vi "configureConnectorPane.vi"(8 "error in (no error)":errorcluster, 11 "PolymorphicInstance in":refnum<class "PolymorphicInstance.lvclass">) -> (0 "error out":errorcluster, 3 "PolymorphicInstance out":refnum<class "PolymorphicInstance.lvclass">)   [LabVIEW 2012, in "PolymorphicInstance.lvclass"]
uses:
  PolymorphicInstance.lvclass
  PolymorphicInstance.lvclass/PolymorphicInstance.ctl
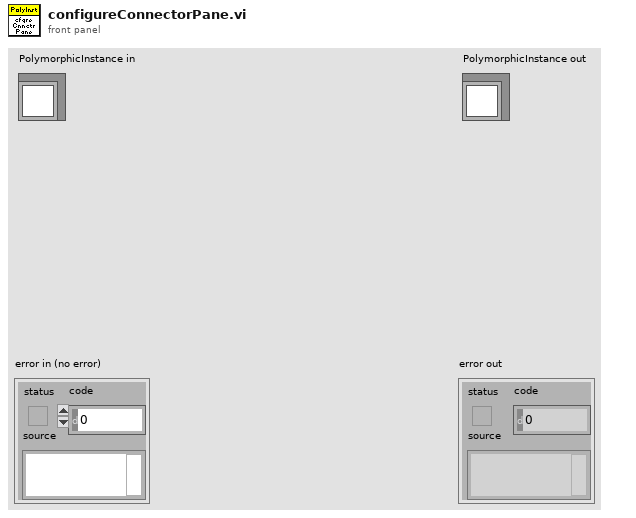
[diagram p1: front panel]
types:
  T1 = enum16{"Invalid Wire Rule", "Required", "Recommended", "Optional", "Dynamic Dispatch"}
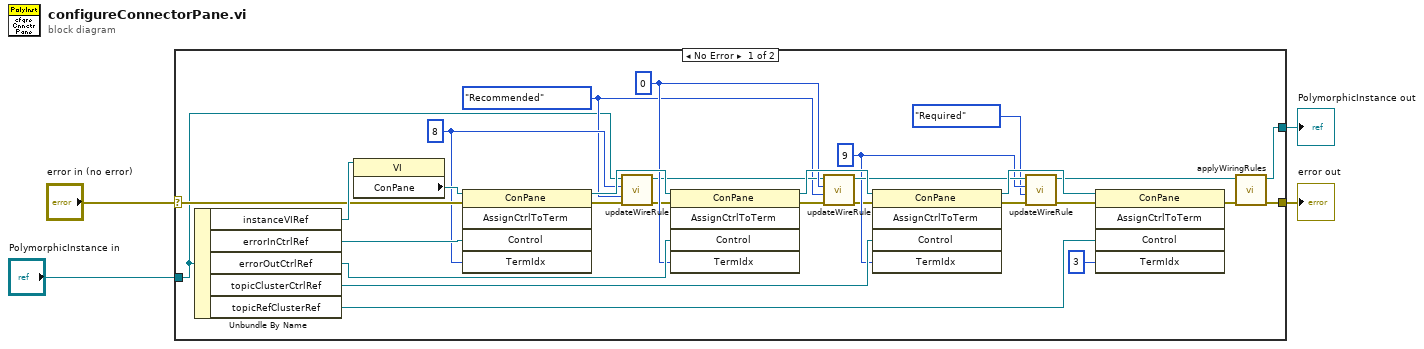
[diagram p0: block diagram]
diagram:
  n1 = case shown="No Error" "error in (no error)" {
    selector: "error in (no error)" -> [w30 w35]
    tunnel: [w14 w35] -> w3
    tunnel: [w12 w34] -> w1
    tunnel: "PolymorphicInstance in" -> [w15 w34]
    frame No Error {
      w19 = T1."Recommended" ("Wire Rule")
      w17 = u32 9 ("Terminal Index")
      w21 = u32 0 ("Terminal Index")
      w22 = u32 8 ("Terminal Index")
      n2 = Unbundle By Name(w15) -> ("instanceVIRef"=w33:refnum<vi>, "errorInCtrlRef"=w31:refnum<vi>, "errorOutCtrlRef"=w29:refnum<vi>, "topicClusterCtrlRef"=w24:refnum<vi>, "topicRefClusterRef"=w23:refnum<vi>)
      n3 = property class="VI"(reference=w33) -> ("ConPane"=w32:refnum<vi>)  [unwired: 1 in, 2 out]
      n4 = invoke class="ConPane" method="AssignCtrlToTerm"(reference=w32, error in=w30, "Control"=w31, "TermIdx"=w22) -> (reference out=w28:refnum<vi>, error out=w11:errorcluster)  [unwired: 1 in, 3 out]
      n5 = call "updateWireRule.vi"("error in (no error)"=w11, "Wire Rule"=w19, "terminalIndex"=w22, "PolymorphicInstance in"=w15) -> ("error out"=w10:errorcluster, "PolymorphicInstance out"=w20:refnum<class "PolymorphicInstance.lvclass">)  [unwired: 6 in]
      n6 = invoke class="ConPane" method="AssignCtrlToTerm"(reference=w28, error in=w10, "Control"=w29, "TermIdx"=w21) -> (reference out=w26:refnum<vi>, error out=w9:errorcluster)  [unwired: 1 in, 3 out]
      n7 = call "updateWireRule.vi"("error in (no error)"=w9, "Wire Rule"=w19, "terminalIndex"=w21, "PolymorphicInstance in"=w20) -> ("error out"=w8:errorcluster, "PolymorphicInstance out"=w18:refnum<class "PolymorphicInstance.lvclass">)  [unwired: 6 in]
      n8 = invoke class="ConPane" method="AssignCtrlToTerm"(reference=w26, error in=w8, "Control"=w24, "TermIdx"=w17) -> (reference out=w25:refnum<vi>, error out=w7:errorcluster)  [unwired: 1 in, 3 out]
      n9 = call "updateWireRule.vi"("error in (no error)"=w7, "Wire Rule"=T1."Required", "terminalIndex"=w17, "PolymorphicInstance in"=w18) -> ("error out"=w6:errorcluster, "PolymorphicInstance out"=w13:refnum<class "PolymorphicInstance.lvclass">)  [unwired: 6 in]
      n10 = invoke class="ConPane" method="AssignCtrlToTerm"(reference=w25, error in=w6, "Control"=w23, "TermIdx"=u32 3 ("Terminal Index")) -> (error out=w5:errorcluster)  [unwired: 1 in, 4 out]
      n11 = call "applyWiringRules.vi"("error in (no error)"=w5, "PolymorphicInstance in"=w13) -> ("error out"=w14:errorcluster, "PolymorphicInstance out"=w12:refnum<class "PolymorphicInstance.lvclass">)  [unwired: 8 in]
    }
    frame Error {
    }
  }
  "error out" <- w3
  "PolymorphicInstance out" <- w1
